vi "TM좌표변환.vi"(2 "lon":dbl format="%#.8g", 3 "lat":dbl format="%#.8g") -> (0 "Y_TM":dbl format="%#.8g", 1 "X_TM":dbl format="%#.8g")   [LabVIEW 2016]
uses:
  <vilib>/imath/engines/lvmath2/RunTimeEngine/Managers/WorkSpace/UID Generator.vi
  <vilib>/imath/engines/lvmath2/RunTimeEngine/RunTimeType/NIMS_RunTimeType_From StrictType (excl LVString).vi
  <instcachedir>/0/NIMS_RunTimeType_From StrictType (excl LVString)_BBF44FB49F834B71AF7A14CCEDF8BECD.lvgen/NIMS_RunTimeType_From StrictType (excl LVString)_BBF44FB49F834B71AF7A14CCEDF8BECD_000.vi
  <vilib>/imath/engines/lvmath2/RunTimeEngine/LocalVariableDefStatement/MC_LocalVariableDefStatement_Display.vi
  <vilib>/imath/engines/lvmath2/RunTimeEngine/BuiltInFunctions/deg_to_rad/NIMS_deg_to_rad.vi
  <instcachedir>/0/NIMS_deg_to_rad_4A81D684CE8D4DD79924F5AB74D756E1.lvgen/NIMS_deg_to_rad_4A81D684CE8D4DD79924F5AB74D756E1_001.vi
  <vilib>/imath/engines/lvmath2/RunTimeEngine/ArithmeticOperatorToken/NIMS_ArithmeticOperator_power(S).vi
  <instcachedir>/0/NIMS_ArithmeticOperator_power(S)_1E6AB98FD36540B9B758A69A385A1B47.lvgen/NIMS_ArithmeticOperator_power(S)_1E6AB98FD36540B9B758A69A385A1B47_014.vi
  <vilib>/imathl/engines/lvmath/Functions/Error Handling/Create Error.vi
  <vilib>/imath/engines/lvmath2/RunTimeEngine/ArithmeticOperatorToken/NIMS_ArithmeticOperator_multmx(M,CV)-internal.vi
  <instcachedir>/0/NIMS_ArithmeticOperator_multmx(M,CV)-internal_14A0C3390E0F41A88768D45F6518085A.lvgen/NIMS_ArithmeticOperator_multmx(M,CV)-internal_14A0C3390E0F41A88768D45F6518085A_002.vi
  <vilib>/imath/engines/lvmath2/RunTimeEngine/IndexRead/NIMS V(S).vi
  <instcachedir>/0/NIMS V(S)_0488751826AF41519A22953C041130DC.lvgen/NIMS V(S)_0488751826AF41519A22953C041130DC_003.vi
  <vilib>/imath/engines/lvmath2/RunTimeEngine/Managers/SymbolTable/Clear UID.vi
  <vilib>/imath/engines/lvmath2/RunTimeEngine/NodeEndStatement/NIMS_NodeEndStatement_Output.vi
  <instcachedir>/0/NIMS_NodeEndStatement_Output_53EC0D466D134D7ABD903AC30B43404B.lvgen/NIMS_NodeEndStatement_Output_53EC0D466D134D7ABD903AC30B43404B_009.vi
  <vilib>/imath/engines/lvmath2/RunTimeEngine/ErrorHandling/NIMS_Finalize Error.vi
  <vilib>/imath/engines/lvmath2/RunTimeEngine/Managers/SymbolTable/NIMS_WorkSpace.lvlib
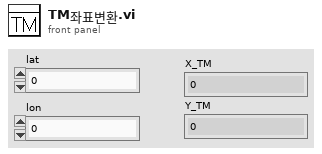
[diagram p1: front panel]
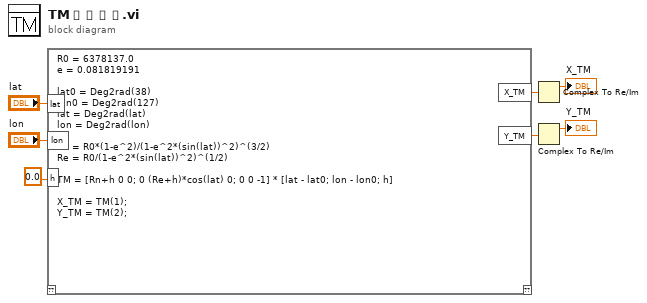
[diagram p0: block diagram]
diagram:
  n1 = mathscript code="R0 = 6378137.0\ne = 0.081819191\n\nlat0 = Deg2rad(38)\nlon0 = Deg2rad(127)\nlat = Deg2rad(lat)\nlon = Deg2rad(lon)\n\nRn = R0*(1-e^2)/(1-e^2*(sin(lat))^2)^(3/2)\nRe = R0/(1-e^2*(sin(lat))^2)^(1/2)\n\nTM = [Rn+h 0 0; 0 (Re+h)*cos(lat) 0; 0 0 -1] * [lat - lat0; lon - lon0; h]\n\nX_TM = TM(1);\nY_TM = TM(2);"("lat"="lat", "h"=0.0, "lon"="lon") -> ("Y_TM"=w3:cdb, "X_TM"=w4:cdb)  [unwired: 1 in, 1 out]
  n2 = Complex To Re/Im(x + iy=w4) -> (x=→"X_TM":dbl)  [unwired: 1 out]
  n3 = Complex To Re/Im(x + iy=w3) -> (x=→"Y_TM":dbl)  [unwired: 1 out]
